vi "Division.vi"() -> ()   [LabVIEW 2014]
panel:
  out "Result":dbl
  in  "Num 2":dbl
  in  "Num 1":dbl
  # "Click          to run"
  # "÷"
  # "="
  # "Division"
  # "The goal of this exercise is simple. Make a calculator that does division. The challenge is that you cannot use the built in divide (or multiply) functions from the mathematics pallete. Only addition and subtraction.\nFurthermore, you must calculate the quotient to four decimal places.\nI would suggest using strings to keep tract of the decimal point. You don't have to use this. But if you are creative enough to come up with your own method of doing this, that's even better."
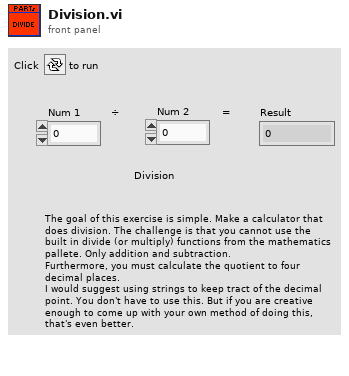
[diagram p1: front panel]
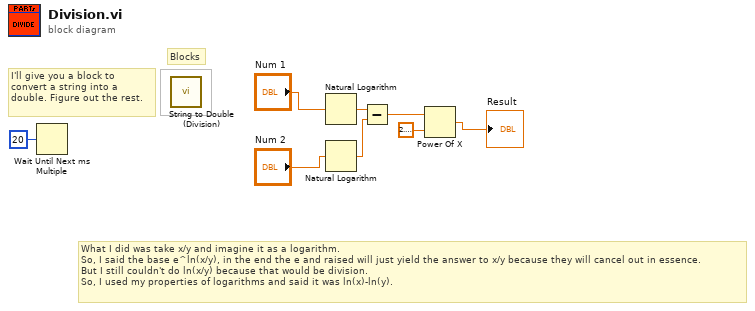
[diagram p0: block diagram]
diagram:
  # "What I did was take x/y and imagine it as a logarithm.\nSo, I said the base e^ln(x/y), in the end the e and raised will just yield the answer to x/y because they will cancel out in essence.\nBut I still couldn't do ln(x/y) because that would be division.\nSo, I used my properties of logarithms and said it was ln(x)-ln(y)."
  # "I'll give you a block to convert a string into a double. Figure out the rest."
  # "Blocks"
  n1 = Wait Until Next ms Multiple(millisecond multiple=u32 20) -> ()  [unwired: 1 out]
  n2 = call "String to Double (Division).vi"() -> ()  [unwired: 1 in, 1 out]
  n3 = Natural Logarithm(1:"Num 1") -> (0:w5:dbl)
  n4 = Natural Logarithm(1:"Num 2") -> (0:w4:dbl)
  n5 = Subtract(x=w5, y=w4) -> (x-y=w6:dbl)
  n6 = Power Of X(1:2.718281828459045, 2:w6) -> (0:→"Result":dbl)
